vi "Project3.vi"() -> ()   [LabVIEW 2024]
panel:
  out "AtoD":dbl format="%01.0f"
  in  "stop":bool
  out "Low FLow":bool
  out "Flow Rate, unit":dbl(knob) scale=0.0..10.0 scale format="%01.2f"
  out "head, M":dbl(slide) scale=0.0..15.0 scale format="%0#1.2f"
  out "Level, M":dbl(slide) scale=0.0..7.0 scale format="%01.2f"
  out "Pressuer, KPA":dbl(knob) scale=0.0..65.0 scale format="%0#1.2f"
  out "Amp, ma":dbl(knob) scale=0.0..25.0 scale format="%0#1.2f"
  out "SCC, V":dbl(knob) scale=0.0..10.0 scale format="%1.3f"
  out "AtoD":i16 format="%1x"
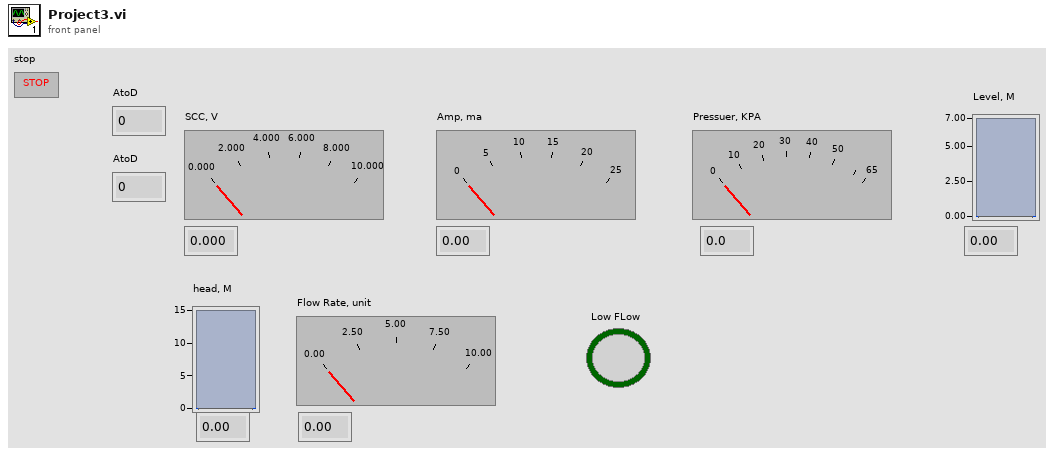
[diagram p1: front panel]
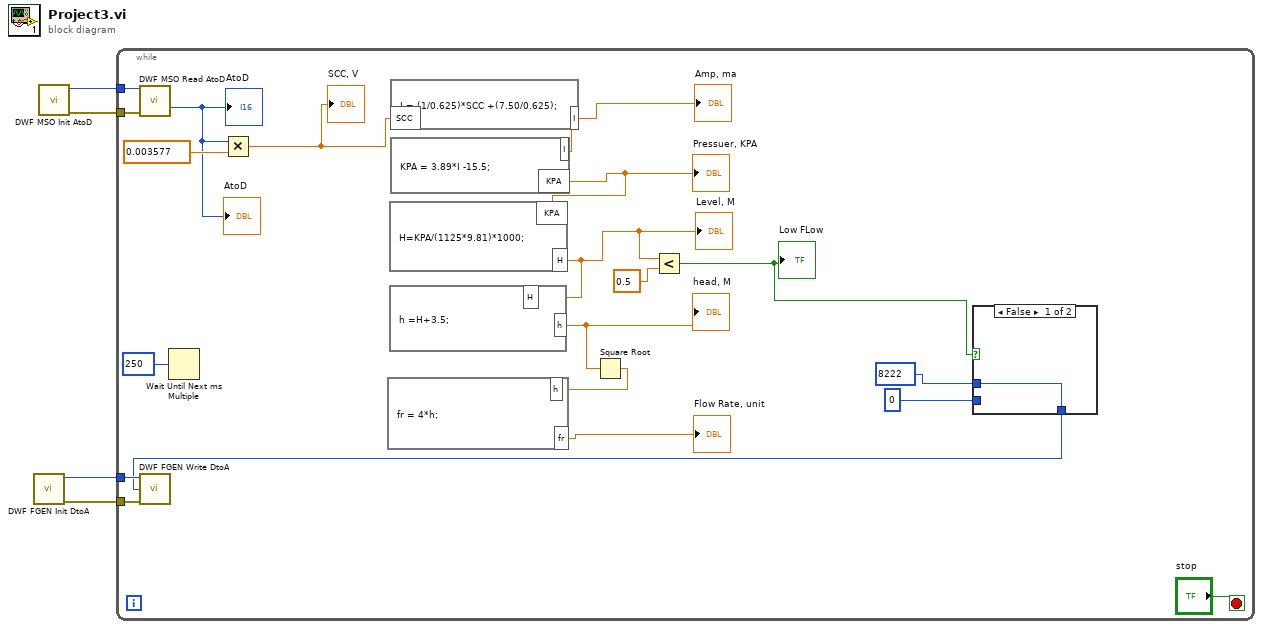
[diagram p0: block diagram]
diagram:
  n1 = call "DWF FGEN Init DtoA.vi"() -> ("Error Out"=w1:errorcluster, "Instrument Handle Out"=w2:u32)  [unwired: 10 in]
  n2 = call "DWF MSO Init AtoD.vi"() -> ("Error Out"=w3:errorcluster, "Instrument Handle Out"=w4:u32)  [unwired: 10 in]
  n3 = while {
    tunnel: w4 -> [w23]
    tunnel: w3 -> [w22]
    tunnel: w2 -> [w14]
    tunnel: w1 -> [w13]
    stop <- "stop" stop-if-true
    n4 = call "DWF MSO Read AtoD.vi"("Instrument Handle In AtoD"=w23, "Error In"=w22) -> ("AtoD"=w5:i16)  [unwired: 12 in, 1 out]
    "AtoD" <- w5
    "AtoD" <- w5
    n5 = Wait Until Next ms Multiple(millisecond multiple=250) -> ()  [unwired: 1 out]
    n6 = Multiply(x=w5, y=0.003577) -> (x*y=w20:dbl)
    "SCC, V" <- w20
    n7 = formula code="I = (1/0.625)*SCC +(7.50/0.625);"("SCC"=w20) -> ("I"=w19:dbl)
    "Amp, ma" <- w19
    n8 = formula code="KPA = 3.89*I -15.5;"("I"=w19) -> ("KPA"=w7:dbl)
    "Pressuer, KPA" <- w7
    n9 = formula code="H=KPA/(1125*9.81)*1000;"("KPA"=w7) -> ("H"=w6:dbl)
    "Level, M" <- w6
    n10 = formula code="h =H+3.5;"("H"=w6) -> ("h"=w18:dbl)
    "head, M" <- w18
    n11 = Square Root(x=w18) -> (sqrt(x)=w17:dbl)
    n12 = formula code="fr = 4*h;"("h"=w17) -> ("fr"=→"Flow Rate, unit":dbl)
    n13 = Less?(x=w6, y=0.5) -> (x < y?=w12:bool)
    "Low FLow" <- w12
    n14 = case shown="False" w12 {
      tunnel: 8222 -> [w25 _]
      tunnel: 0 -> [_ w26]
      tunnel: [w25 w26] -> w9
      frame False {
      }
      frame True {
      }
    }
    n15 = call "DWF FGEN Write DtoA.vi"("Error In"=w13, "Raw Data"=w9, "Instrument Handle In"=w14) -> ()  [unwired: 1 in, 2 out]
  }
